vi "Initialization VI.vi"(8 "error in (no error)":errorcluster, 10 "Custom XML":string, 11 "Device Item Ref in":T1 format="%.0x") -> (0 "error out":errorcluster, 3 "Device Item Ref out":T1 format="%.0x")   [LabVIEW 2020, in "Ballard MIL-STD-1553 System Explorer.lvlib"]
uses:
  Ballard MIL-STD-1553 System Explorer.lvlib
  <vilib>/NI VeriStand/Custom Device API/Custom Device Item Ref.ctl
  Includes/Ballard MIL-STD-1553 System Explorer.lvlibp/System Explorer/Implementation/Implementation.lvlib
  <vilib>/NI VeriStand/Custom Device API/Custom Device API.lvlib
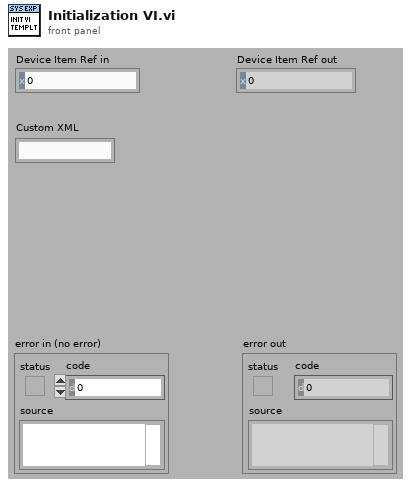
[diagram p1: front panel]
types:
  T1 = typedef "Custom Device API.lvlib/Custom Device Item Ref.ctl" = u64
  T2 = typedef "Ballard MIL-STD-1553 System Explorer.lvlibp/Custom Device API.lvlib/Custom Device Item Ref.ctl" = u64
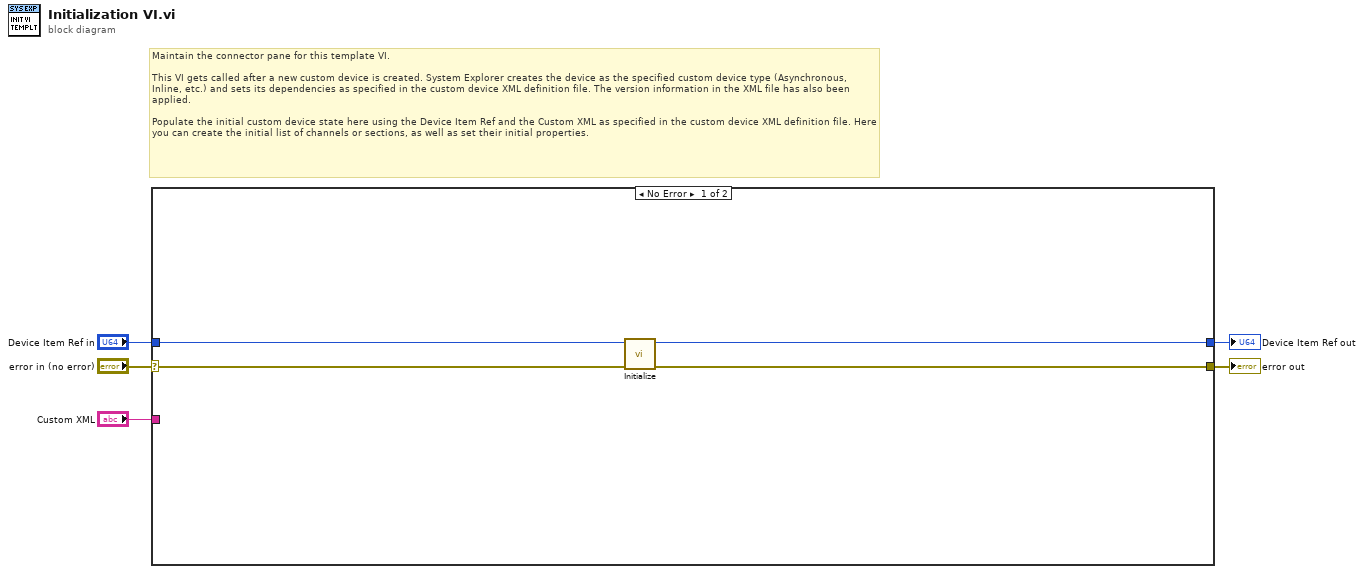
[diagram p0: block diagram]
diagram:
  # "Maintain the connector pane for this template VI.\n\nThis VI gets called after a new custom device is created. System Explorer creates the device as the specified custom device type (Asynchronous, Inline, etc.) and sets its dependencies as specified in the custom device XML definition file. The version information in the XML file has also been applied.\n\nPopulate the initial custom device state here using the Device Item Ref and the Custom XML as specified in the custom device XML definition file. Here you can create the initial list of channels or sections, as well as set their initial properties."
  n1 = case shown="No Error" "error in (no error)" {
    selector: "error in (no error)" -> [w8 w11]
    tunnel: [w7 w11] -> w5
    tunnel: [w6 w10] -> w3
    tunnel: "Device Item Ref in" -> [w9 w10]
    tunnel: "Custom XML" -> [_ _]
    frame No Error {
      n2 = call "Initialize.vi"("error in (no error)"=w8, "Device Item Ref in"=w9) -> ("error out"=w7:errorcluster, "Device Item Ref out"=w6:T2)  [unwired: 8 in]
    }
    frame Error {
    }
  }
  "error out" <- w5
  "Device Item Ref out" <- w3
